vi "Toolkit - Find All Clusters.vi"() -> ()   [LabVIEW 2017]
doc: "Finds all of the clusters in the block diagram and front panel of a VI using VI scripting and the ACE Toolkit API."
uses:
  Toolkit/Toolkit.lvlib
panel:
  out "Cluster Count":i32
  # "Overview: Demonstrates finding all clusters in a VI using VI scripting the ACE toolkit\nInstructions:\n1. Run this VI"
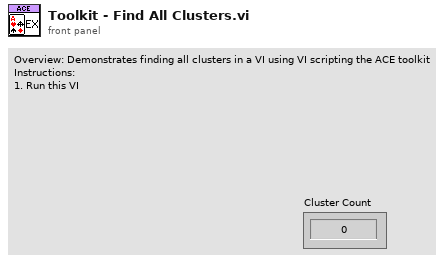
[diagram p1: front panel]
types:
  T1 = enum32{"Invalid", "Standard", "Closed", "Hidden", "Minimized", "Maximized"}
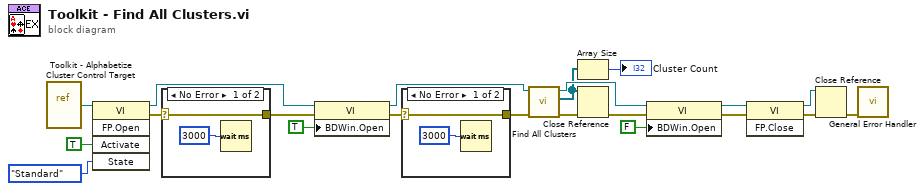
[diagram p0: block diagram]
diagram:
  n1 = vi-ref "Toolkit - Alphabetize Cluster Control Target.vi"() -> (w12:refnum<vi>)
  n2 = invoke class="VI" method="FP.Open"(reference=w12, "Activate"=TRUE ("Activate?"), "State"=T1."Standard") -> (reference out=w15:refnum<vi>, error out=w3:errorcluster)  [unwired: 2 in, 3 out]
  n3 = case shown="No Error" w3 {
    selector: w3 -> [w23 w24]
    tunnel: [w23 w24] -> w2
    frame No Error {
      n4 = Wait (ms)(milliseconds to wait=u32 3000) -> ()  [unwired: 1 out]
    }
    frame Error {
    }
  }
  n5 = property class="VI"(reference=w15, error in=w2, "BDWin.Open"=TRUE ("Block Diagram Window:Open")) -> (reference out=w14:refnum<vi>, error out=w13:errorcluster)
  n6 = case shown="No Error" w13 {
    selector: w13 -> [w26 w27]
    tunnel: [w26 w27] -> w18
    frame No Error {
      n7 = Wait (ms)(milliseconds to wait=u32 3000) -> ()  [unwired: 1 out]
    }
    frame Error {
    }
  }
  n8 = call "Find All Clusters.vi"("Error In"=w18, "VI In"=w14) -> ("Error Out"=w5:errorcluster, "Clusters"=w6:refnum<vi>[], "VI Out"=w10:refnum<vi>)  [unwired: 7 in]
  n9 = Array Size(array=w6) -> (size(s)=→"Cluster Count":i32)
  n10 = Close Reference(reference=w6, error in (no error)=w5) -> (error out=w1:errorcluster)
  n11 = property class="VI"(reference=w10, error in=w1, "BDWin.Open"=FALSE ("Block Diagram Window:Open")) -> (reference out=w9:refnum<vi>, error out=w8:errorcluster)
  n12 = invoke class="VI" method="FP.Close"(reference=w9, error in=w8) -> (reference out=w17:refnum<vi>, error out=w16:errorcluster)  [unwired: 1 in, 1 out]
  n13 = Close Reference(reference=w17, error in (no error)=w16) -> (error out=w21:errorcluster)
  n14 = call <vilib>:"General Error Handler.vi"("error in (no error)"=w21) -> ()  [unwired: 10 in, 5 out]
